vi "Read Faulted State.vi"(11 "statemachine in":refnum<class "statemachine.lvclass">) -> (2 "Faulted State":refnum<class "state.lvclass">, 3 "statemachine out":refnum<class "statemachine.lvclass">)   [LabVIEW 2020, in "eos.lvlib" / "statemachine.lvclass"]
uses:
  statemachine.lvclass
  interfaces/state/state.lvclass
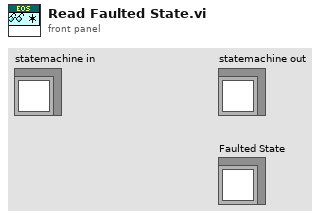
[diagram p1: front panel]
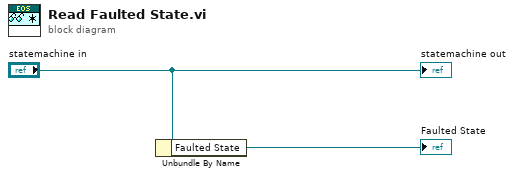
[diagram p0: block diagram]
diagram:
  n1 = Unbundle By Name("statemachine in") -> ("Faulted State"=→"Faulted State":refnum<class "state.lvclass">)
  "statemachine out" <- "statemachine in"
